vi "DAQmx Read (Counter Pulse Ticks 1Chan 1Samp).vi"(0 "task/channels in":refnum<k21>, 9 "timeout":dbl=10.0 format="%0.2f", 11 "error in":errorcluster) -> (4 "task out":refnum<k21>, 6 "high ticks":u32, 8 "low ticks":u32, 15 "error out":errorcluster)   [LabVIEW 2020]
doc: "Reads a single pair of pulse high and low tick counts from a counter input task."
uses:
  nilvaiu.dll
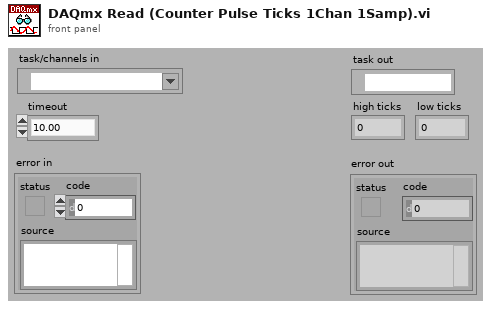
[diagram p1: front panel]
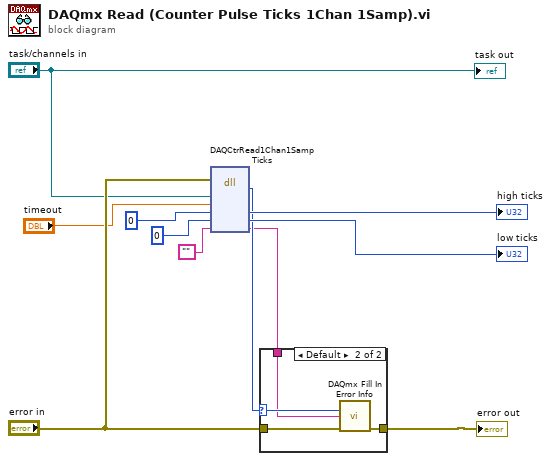
[diagram p0: block diagram]
diagram:
  n1 = dll-call lib="nilvaiu.*" fn="DAQCtrRead1Chan1SampTicks"(error in="error in", "taskID"="task/channels in", "timeout"="timeout", "highTicks"=u32 0, "lowTicks"=u32 0, "extendedErrorInfo"="") -> ("return type"=w5:i32, "highTicks"=→"high ticks":u32, "lowTicks"=→"low ticks":u32, "extendedErrorInfo"=w3:string)  [unwired: 3 in, 3 out]
  n2 = case shown="Default" w5 {
    selector: w5 -> [_ w14]
    tunnel: "error in" -> [w12 w16]
    tunnel: [w12 w15] -> w10
    tunnel: w3 -> [_ w13]
    frame 0 {
    }
    frame Default {
      n3 = call "DAQmx Fill In Error Info.vi"("status code"=w14, "extended error info"=w13, "error in"=w16) -> ("error out"=w15:errorcluster)  [unwired: 1 in, 11 out]
    }
  }
  "error out" <- w10
  "task out" <- "task/channels in"
